vi "1.vi"() -> ()   [LabVIEW 2014]
doc: "When installed on computers on a LAN this vi will allow people on different computers to communicate with each other through the LAN\n\nContact:\nfelannan@yahoo.com"
uses:
  <vilib>/sound/lvsound.llb/Sound Format.ctl
panel:
  out "Remote Address":string
  out "C":bool
  in  "Disconnect":bool
  in  "?":enum32{"Call", "Settings"}(tab)
  in  "Connect":bool
  in  "Address":string="127.0.0.1"
  in  "Mic":u32
  in  "Speaker":u32
  in  "Accept":bool
  out "TF":bool caption="Disconnected"
  in  "Typecast":u8[](array[numeric])
  out "connection ID":refnum<k5>
  # "V   IP"
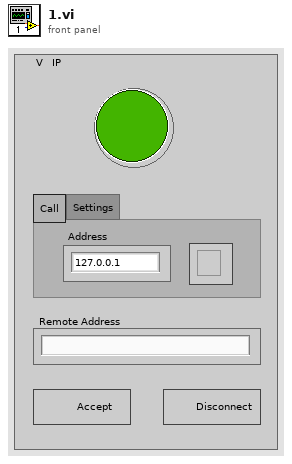
[diagram p1: front panel]
types:
  T1 = typedef "Sound Format.ctl" = cluster{"sound quality":enum16{"mono", "stereo"}, "rate":enum16{"11025", "22050", "44100", "8000"}, "bits per sample":enum16{"8 bit", "16 bit"}}
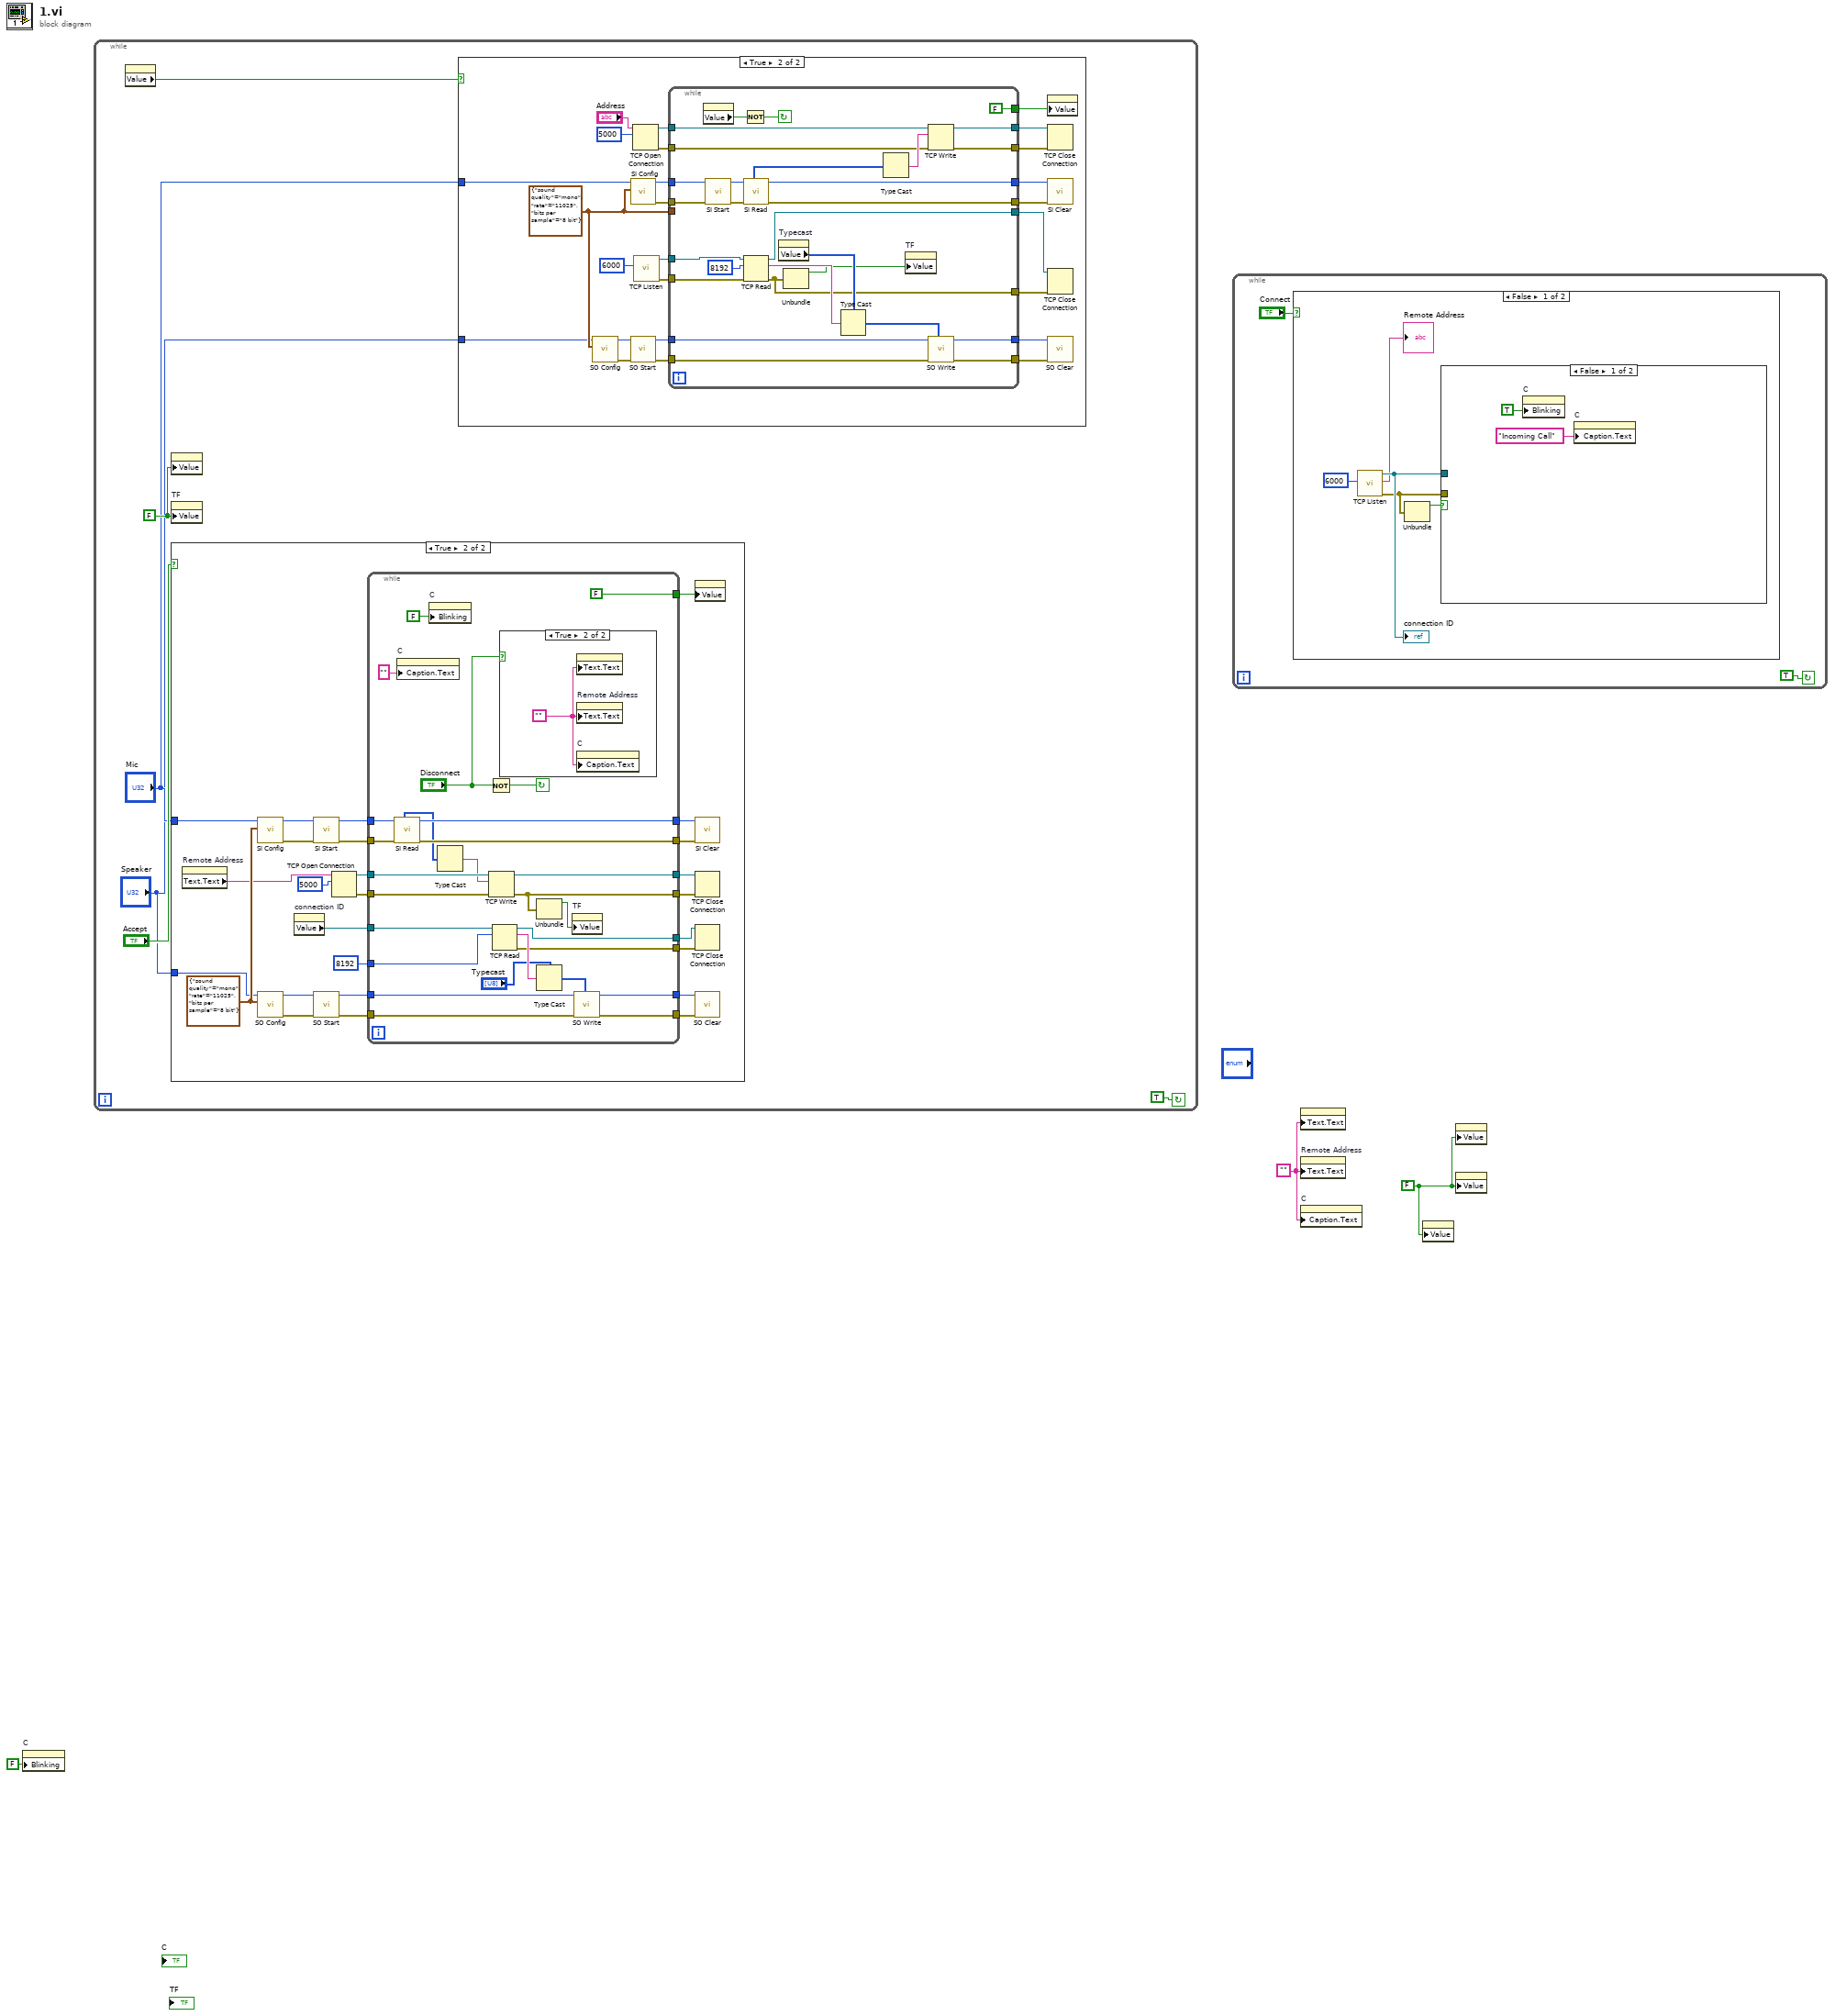
[diagram p0: block diagram]
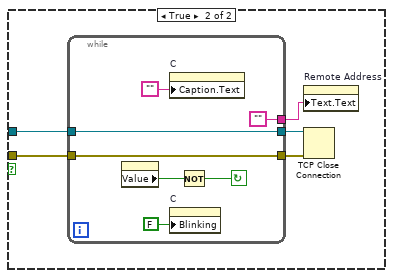
[diagram p5: hidden frame]
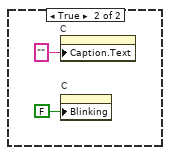
[diagram p6: hidden frame]
diagram:
  w1 = "" ("Caption.Text")
  w2 = FALSE ("Call")
  n1 = property on="C" class="Bool (strict)"("Blinking"=FALSE) -> ()  [unwired: 2 in, 2 out]
  n2 = while {
    stop <- TRUE continue-if-true
    w6 = FALSE
    n3 = property class="Bool (strict)"() -> ("Value"=w9:bool)  [unwired: 2 in, 2 out]
    n4 = property class="Bool (strict)"("Value"=w6) -> ()  [unwired: 2 in, 2 out]
    n5 = property on="TF" class="Bool (strict)"("Value"=w6) -> ()  [unwired: 2 in, 2 out]
    n6 = case shown="True" "Accept" {
      tunnel: "Mic" -> [_ w12]
      tunnel: "Speaker" -> [_ w11]
      frame False {
      }
      frame True {
        w13 = T1 {"sound quality"=enum."mono", "rate"=enum."11025", "bits per sample"=enum."8 bit"} ("sound format")
        n7 = property on="Remote Address" class="Str"() -> ("Text.Text"=w10:string)  [unwired: 2 in, 2 out]
        n8 = call <vilib>:"SI Config.vi"("sound format"=w13, "device (0)"=w12) -> ("error out"=w26:errorcluster, "task ID out"=w27:u32)  [unwired: 8 in]
        n9 = call <vilib>:"SO Config.vi"("sound format"=w13, "device (0)"=w11) -> ("error out"=w32:errorcluster, "task ID out"=w33:u32)  [unwired: 8 in]
        n10 = property on="connection ID" class="Ref (strict)"() -> ("Value"=w35:refnum<k5>)  [unwired: 2 in, 2 out]
        n11 = call <vilib>:"SI Start.vi"("error in (no error)"=w26, "task ID in"=w27) -> ("error out"=w24:errorcluster, "task ID out"=w25:u32)  [unwired: 8 in]
        n12 = call <vilib>:"SO Start.vi"("error in (no error)"=w32, "task ID in"=w33) -> ("error out"=w30:errorcluster, "task ID out"=w31:u32)  [unwired: 8 in]
        n13 = TCP Open Connection(address=w10, remote port or service name=u16 5000 ("remote port")) -> (connection ID=w28:refnum<k5>, error out=w14:errorcluster)  [unwired: 3 in]
        n14 = while {
          tunnel: w35 -> [w62]
          tunnel: 8192 ("bytes to read") -> [w61]
          tunnel: w31 -> [w58]
          tunnel: w30 -> [w57]
          tunnel: w28 -> [w56]
          tunnel: w14 -> [w55]
          tunnel: w25 -> [w54]
          tunnel: w24 -> [w53]
          tunnel: [w50] -> w23
          tunnel: [w49] -> w22
          tunnel: [w48] -> w21
          tunnel: [w40] -> w20
          tunnel: [w47] -> w19
          tunnel: [w46] -> w18
          tunnel: [w45] -> w17
          tunnel: [w44] -> w16
          tunnel: [FALSE] -> w15
          stop <- w51 continue-if-true
          n15 = call <vilib>:"SI Read.vi"("error in (no error)"=w53, "task ID in"=w54) -> ("error out"=w46:errorcluster, "task ID out"=w47:u32, "mono 8-bit"=w42:u8[])  [unwired: 4 in, 3 out]
          n16 = property on="C" class="Bool (strict)"("Caption.Text"="") -> ()  [unwired: 2 in, 2 out]
          n17 = property on="C" class="Bool (strict)"("Blinking"=FALSE) -> ()  [unwired: 2 in, 2 out]
          n18 = Type Cast(x=w42) -> (*(type *) &x=w52:string)  [unwired: 1 in]
          n19 = Not(x="Disconnect") -> (.not. x?=w51:bool)
          n20 = TCP Write(connection ID=w56, data in=w52, error in (no error)=w55) -> (connection ID out=w48:refnum<k5>, error out=w40:errorcluster)  [unwired: 1 in, 1 out]
          n21 = TCP Read(connection ID=w62, bytes to read=w61) -> (connection ID out=w50:refnum<k5>, data out=w60:string, error out=w49:errorcluster)  [unwired: 3 in]
          n22 = case shown="True" "Disconnect" {
            frame False {
            }
            frame True {
              w63 = "" ("Caption.Text")
              n23 = property class="Str"("Text.Text"=w63) -> ()  [unwired: 2 in, 2 out]
              n24 = property on="Remote Address" class="Str"("Text.Text"=w63) -> ()  [unwired: 2 in, 2 out]
              n25 = property on="C" class="Bool (strict)"("Caption.Text"=w63) -> ()  [unwired: 2 in, 2 out]
            }
          }
          n26 = Unbundle(w40) -> ("status"=w39:bool)  [unwired: 2 out]
          n27 = Type Cast(type="Typecast", x=w60) -> (*(type *) &x=w41:u8[])
          n28 = property on="TF" class="Bool (strict)"("Value"=w39) -> ()  [unwired: 2 in, 2 out]
          n29 = call <vilib>:"SO Write.vi"("mono 8-bit"=w41, "error in (no error)"=w57, "task ID in"=w58) -> ("error out"=w44:errorcluster, "task ID out"=w45:u32)  [unwired: 7 in]
        }
        n30 = property class="Bool (strict)"("Value"=w15) -> ()  [unwired: 2 in, 2 out]
        n31 = call <vilib>:"SI Clear.vi"("error in (no error)"=w18, "task ID in"=w19) -> ()  [unwired: 9 in, 1 out]
        n32 = TCP Close Connection(connection ID=w21, error in (no error)=w20) -> ()  [unwired: 1 in, 2 out]
        n33 = TCP Close Connection(connection ID=w23, error in (no error)=w22) -> ()  [unwired: 1 in, 2 out]
        n34 = call <vilib>:"SO Clear.vi"("error in (no error)"=w16, "task ID in"=w17) -> ()  [unwired: 9 in, 1 out]
      }
    }
    n35 = case shown="True" w9 {
      tunnel: "Mic" -> [_ w65]
      tunnel: "Speaker" -> [_ w64]
      frame False {
      }
      frame True {
        w88 = T1 {"sound quality"=enum."mono", "rate"=enum."11025", "bits per sample"=enum."8 bit"}
        n36 = call <vilib>:"SO Config.vi"("sound format"=w88, "device (0)"=w64) -> ("error out"=w79:errorcluster, "task ID out"=w80:u32)  [unwired: 8 in]
        n37 = call <vilib>:"SI Config.vi"("sound format"=w88, "device (0)"=w65) -> ("error out"=w66:errorcluster, "task ID out"=w67:u32)  [unwired: 8 in]
        n38 = call <vilib>:"SO Start.vi"("error in (no error)"=w79, "task ID in"=w80) -> ("error out"=w77:errorcluster, "task ID out"=w78:u32)  [unwired: 8 in]
        n39 = TCP Open Connection(address="Address", remote port or service name=u16 5000 ("remote port")) -> (connection ID=w85:refnum<k5>, error out=w84:errorcluster)  [unwired: 3 in]
        n40 = call <vilib>:"TCP Listen.vi"("port"=6000) -> ("error out"=w81:errorcluster, "connection ID"=w82:refnum<k5>)  [unwired: 6 in, 3 out]
        n41 = while {
          tunnel: w88 -> [_]
          tunnel: w85 -> [w114]
          tunnel: w84 -> [w113]
          tunnel: w82 -> [w112]
          tunnel: w81 -> [w111]
          tunnel: w78 -> [w108]
          tunnel: w77 -> [w107]
          tunnel: [w104] -> w76
          tunnel: [w103] -> w75
          tunnel: [w102] -> w74
          tunnel: [w91] -> w73
          tunnel: [w100] -> w72
          tunnel: [w99] -> w71
          tunnel: [w98] -> w70
          tunnel: [w97] -> w69
          tunnel: [FALSE] -> w68
          tunnel: w67 -> [w95]
          tunnel: w66 -> [w94]
          stop <- w105 continue-if-true
          n42 = property class="Bool (strict)"() -> ("Value"=w106:bool)  [unwired: 2 in, 2 out]
          n43 = call <vilib>:"SI Start.vi"("error in (no error)"=w94, "task ID in"=w95) -> ("error out"=w92:errorcluster, "task ID out"=w93:u32)  [unwired: 8 in]
          n44 = Not(x=w106) -> (.not. x?=w105:bool)
          n45 = call <vilib>:"SI Read.vi"("error in (no error)"=w92, "task ID in"=w93) -> ("error out"=w99:errorcluster, "task ID out"=w100:u32, "mono 8-bit"=w115:u8[])  [unwired: 4 in, 3 out]
          n46 = TCP Read(connection ID=w112, bytes to read=8192, error in (no error)=w111) -> (connection ID out=w102:refnum<k5>, data out=w110:string, error out=w91:errorcluster)  [unwired: 2 in]
          n47 = property on="Typecast" class="Arr (strict)"() -> ("Value"=w109:u8[])  [unwired: 2 in, 2 out]
          n48 = Unbundle(w91) -> ("status"=w90:bool)  [unwired: 2 out]
          n49 = Type Cast(type=w109, x=w110) -> (*(type *) &x=w89:u8[])
          n50 = Type Cast(x=w115) -> (*(type *) &x=w116:string)  [unwired: 1 in]
          n51 = property on="TF" class="Bool (strict)"("Value"=w90) -> ()  [unwired: 2 in, 2 out]
          n52 = TCP Write(connection ID=w114, data in=w116, error in (no error)=w113) -> (connection ID out=w104:refnum<k5>, error out=w103:errorcluster)  [unwired: 1 in, 1 out]
          n53 = call <vilib>:"SO Write.vi"("mono 8-bit"=w89, "error in (no error)"=w107, "task ID in"=w108) -> ("error out"=w97:errorcluster, "task ID out"=w98:u32)  [unwired: 7 in]
        }
        n54 = property class="Bool (strict)"("Value"=w68) -> ()  [unwired: 2 in, 2 out]
        n55 = TCP Close Connection(connection ID=w76, error in (no error)=w75) -> ()  [unwired: 1 in, 2 out]
        n56 = call <vilib>:"SI Clear.vi"("error in (no error)"=w71, "task ID in"=w72) -> ()  [unwired: 9 in, 1 out]
        n57 = TCP Close Connection(connection ID=w74, error in (no error)=w73) -> ()  [unwired: 1 in, 2 out]
        n58 = call <vilib>:"SO Clear.vi"("error in (no error)"=w69, "task ID in"=w70) -> ()  [unwired: 9 in, 1 out]
      }
    }
  }
  n59 = while {
    stop <- TRUE continue-if-true
    n60 = case shown="False" "Connect" {
      frame False {
        n61 = call <vilib>:"TCP Listen.vi"("port"=u16 6000) -> ("error out"=w120:errorcluster, "remote address"=→"Remote Address":string, "connection ID"=w121:refnum<k5>)  [unwired: 6 in, 2 out]
        "connection ID" <- w121
        n62 = Unbundle(w120) -> ("status"=w122:bool)  [unwired: 2 out]
        n63 = case shown="False" w122 {
          tunnel: w121 -> [_ w130]
          tunnel: w120 -> [_ w128]
          frame False {
            n64 = property on="C" class="Bool (strict)"("Blinking"=TRUE) -> ()  [unwired: 2 in, 2 out]
            n65 = property on="C" class="Bool (strict)"("Caption.Text"="Incoming Call") -> ()  [unwired: 2 in, 2 out]
          }
          frame True {
            n66 = while {
              tunnel: [""] -> w126
              tunnel: w130 -> [w135]
              tunnel: [w135] -> w129
              tunnel: w128 -> [w134]
              tunnel: [w134] -> w127
              stop <- w137 continue-if-true
              n67 = property class="Bool (strict)"() -> ("Value"=w133:bool)  [unwired: 2 in, 2 out]
              n68 = property on="C" class="Bool (strict)"("Caption.Text"="") -> ()  [unwired: 2 in, 2 out]
              n69 = property on="C" class="Bool (strict)"("Blinking"=FALSE) -> ()  [unwired: 2 in, 2 out]
              n70 = Not(x=w133) -> (.not. x?=w137:bool)
            }
            n71 = property on="Remote Address" class="Str"("Text.Text"=w126) -> ()  [unwired: 2 in, 2 out]
            n72 = TCP Close Connection(connection ID=w129, error in (no error)=w127) -> ()  [unwired: 1 in, 2 out]
          }
        }
      }
      frame True {
        n73 = property on="C" class="Bool (strict)"("Caption.Text"="") -> ()  [unwired: 2 in, 2 out]
        n74 = property on="C" class="Bool (strict)"("Blinking"=FALSE) -> ()  [unwired: 2 in, 2 out]
      }
    }
  }
  n75 = property class="Str"("Text.Text"=w1) -> ()  [unwired: 2 in, 2 out]
  n76 = property on="Remote Address" class="Str"("Text.Text"=w1) -> ()  [unwired: 2 in, 2 out]
  n77 = property on="C" class="Bool (strict)"("Caption.Text"=w1) -> ()  [unwired: 2 in, 2 out]
  n78 = property class="Bool (strict)"("Value"=w2) -> ()  [unwired: 2 in, 2 out]
  n79 = property class="Bool (strict)"("Value"=w2) -> ()  [unwired: 2 in, 2 out]
  n80 = property class="Bool (strict)"("Value"=w2) -> ()  [unwired: 2 in, 2 out]
